vi "Weighted_Average.vi"() -> ()   [LabVIEW 2022 SP3]
uses:
  <vilib>/Utility/file.llb/Read Delimited Spreadsheet (DBL).vi
panel:
  out "All Data":dbl[](graph)
  out "Subtract from original signal":dbl(graph)
  out "Weighted Average":dbl(graph)
  out "all rows":dbl[][](array[numeric])
  in  "stop":bool
  in  "file path (dialog if empty)":path
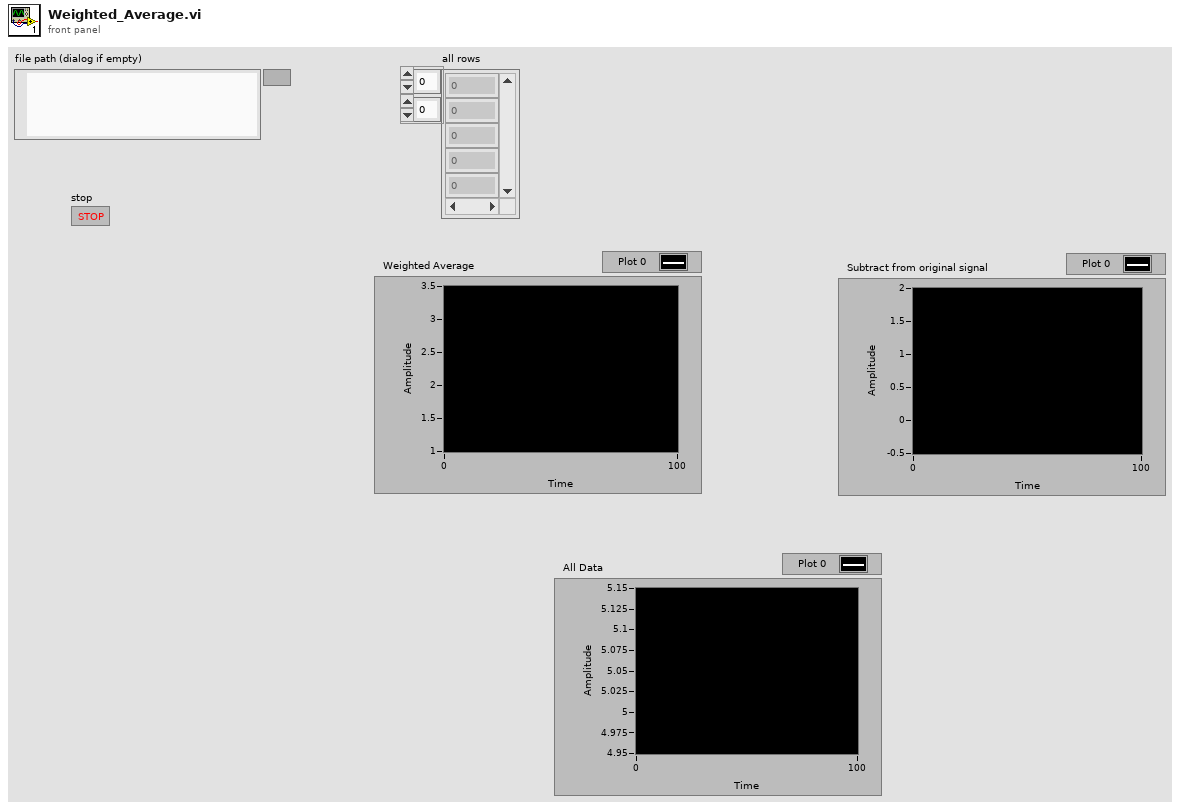
[diagram p1: front panel]
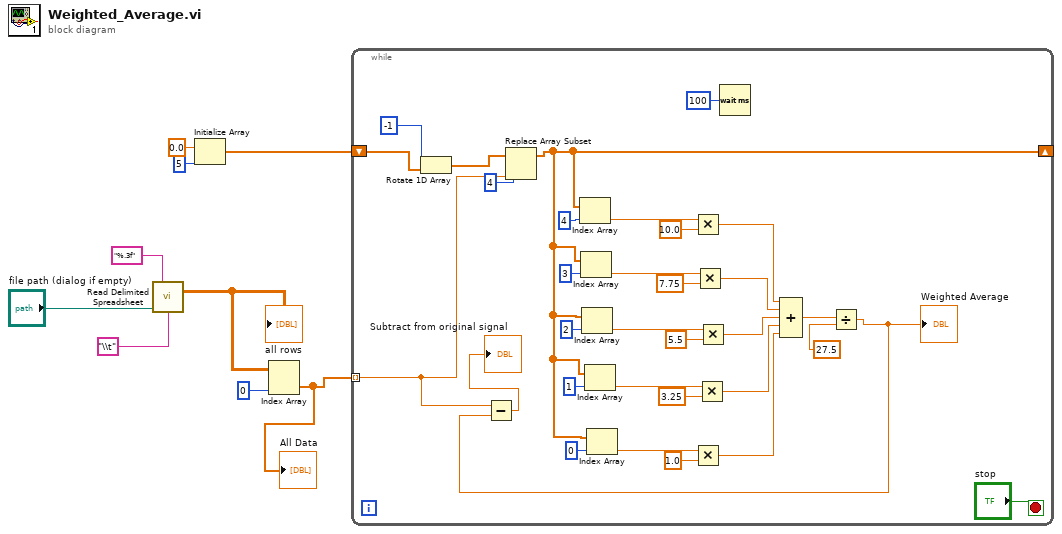
[diagram p0: block diagram]
diagram:
  n1 = call-poly <vilib>:"Read Delimited Spreadsheet.vi"("file path (dialog if empty)"="file path (dialog if empty)", "format (%.3f)"="%.3f", "delimiter (\\t)"="\\t" ("delimiter (\\t)")) -> ("all rows"=w3:dbl[][])  [unwired: 7 in, 5 out]
  "all rows" <- w3
  n2 = Initialize Array "Initialize Array"(0.0 ("element"), 5 ("dimension size")) -> (w4:dbl[])
  n3 = Index Array "Index Array"(array=w3, index (col)=0 ("disabled index (col)")) -> (element=w1:dbl[])  [unwired: 1 in]
  "All Data" <- w1
  n4 = while {
    shift-right: [w34] -> _
    shift-left: w4 -> [w14]
    tunnel: w1 -> [w11] mode=indexing
    stop <- "stop" stop-if-true
    n5 = Rotate 1D Array(1:w14, 2:-1 ("n")) -> (0:w40:dbl[])
    n6 = Replace Array Subset "Replace Array Subset"(array=w40, new element=w11, index=4) -> (w34:dbl[])
    n7 = Index Array "Index Array"(array=w34, index=4) -> (element=w33:dbl)
    n8 = Index Array "Index Array"(array=w34, index=3) -> (element=w32:dbl)
    n9 = Index Array "Index Array"(array=w34, index=2) -> (element=w31:dbl)
    n10 = Index Array "Index Array"(array=w34, index=1) -> (element=w30:dbl)
    n11 = Index Array "Index Array"(array=w34, index=0) -> (element=w29:dbl)
    n12 = Multiply(x=w33, y=10.0) -> (x*y=w23:dbl)
    n13 = Multiply(x=w29, y=1.0) -> (x*y=w19:dbl)
    n14 = Multiply(x=w32, y=7.75) -> (x*y=w22:dbl)
    n15 = Multiply(x=w30, y=3.25) -> (x*y=w20:dbl)
    n16 = Multiply(x=w31, y=5.5) -> (x*y=w21:dbl)
    n17 = Wait (ms)(milliseconds to wait=u32 100) -> ()  [unwired: 1 out]
    n18 = Compound Arithmetic op=ADD(w23, w22, w21, w20, w19) -> (w18:dbl)
    n19 = Divide(x=w18, y=27.5) -> (x/y=w12:dbl)
    "Weighted Average" <- w12
    n20 = Subtract(x=w11, y=w12) -> (x-y=→"Subtract from original signal":dbl)
  }
